vi "GraderMain.vi"   [LabVIEW 2015]
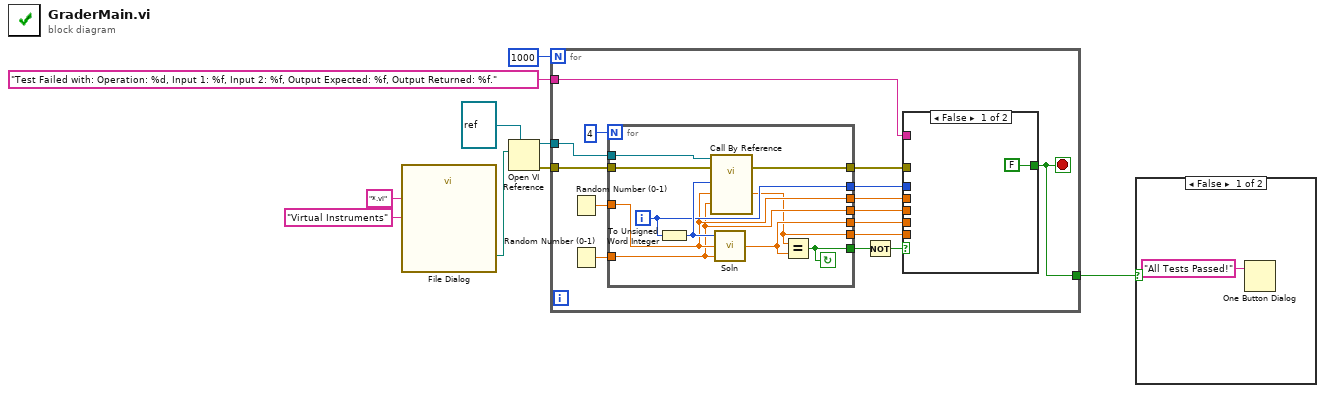
[diagram p0: block diagram]
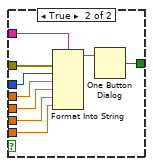
[diagram p3: hidden frame]
diagram:
  n1 = call "File Dialog"("pattern (all files)"="*.vi", "pattern label"="Virtual Instruments") -> ("selected path"=w6:path)  [unwired: 10 in, 3 out]
  n2 = Open VI Reference(type specifier VI Refnum (for type only)=refnum<vi> refnum, vi path=w6) -> (vi reference=w8:refnum<vi>, error out=w9:errorcluster)  [unwired: 4 in]
  n3 = for {
    N: 1000 -> [_]
    tunnel: w9 -> [w24]
    tunnel: w8 -> [w23]
    tunnel: "Test Failed with: Operation: %d, Input 1: %f, Input 2: %f, Output Expected: %f, Output Returned: %f." ("format string") -> [w19]
    tunnel: [w10] -> w3
    stop <- w10 stop-if-true
    n4 = Random Number (0-1)() -> (number: 0 to 1=w21:dbl)
    n5 = Random Number (0-1)() -> (number: 0 to 1=w20:dbl)
    n6 = for {
      N: 4 -> [_]
      tunnel: w24 -> [w44]
      tunnel: w23 -> [w43]
      tunnel: w21 -> [w38]
      tunnel: w20 -> [w37]
      tunnel: [w41] -> w12
      tunnel: [w40] -> w18
      tunnel: [w39] -> w17
      tunnel: [w38] -> w16
      tunnel: [w37] -> w15
      tunnel: [w36] -> w14
      tunnel: [w35] -> w13
      i -> [w39]
      stop <- w41 continue-if-true
      n7 = To Unsigned Word Integer(number=w39) -> (unsigned 16bit integer=w42:u16)
      n8 = call-by-ref "?"(reference=w43, error in=w44, "Input 2"=w37, "Input 1"=w38, "Operation"=w42) -> (error out=w40:errorcluster, "Output"=w35:dbl)  [unwired: 1 out]
      n9 = call "Soln.vi"("Input 2"=w37, "Input 1"=w38, "Operation"=w42) -> ("Output"=w36:dbl)
      n10 = Equal?(x=w35, y=w36) -> (x = y?=w41:bool)
    }
    n11 = Not(x=w12) -> (.not. x?=w11:bool)
    n12 = case shown="False" w11 {
      tunnel: w19 -> [_ w34]
      tunnel: w18 -> [_ w33]
      tunnel: w17 -> [_ w32]
      tunnel: w16 -> [_ w31]
      tunnel: w15 -> [_ w30]
      tunnel: w14 -> [_ w29]
      tunnel: w13 -> [_ w28]
      tunnel: [FALSE ("true") w26] -> w10
      frame False {
      }
      frame True {
        n13 = Format Into String(format string=w34, error in=w33, w32, w31, w30, w29, w28) -> (resulting string=w27:string)  [unwired: 1 in, 1 out]
        n14 = One Button Dialog(message=w27) -> (true=w26:bool)  [unwired: 1 in]
      }
    }
  }
  n15 = case shown="False" w3 {
    frame False {
      n16 = One Button Dialog(message="All Tests Passed!") -> ()  [unwired: 1 in, 1 out]
    }
    frame True {
    }
  }
